vi "Ejercicio_basico_LabView.vi"() -> ()   [LabVIEW 2014]
uses:
  <vilib>/LabVIEW Interface for Arduino/Type Defs/Board Type.ctl
  <vilib>/LabVIEW Interface for Arduino/Type Defs/Pin Mode.ctl
  <vilib>/LabVIEW Interface for Arduino/LabVIEW Interface for Arduino.lvlib
panel:
  in  "VISA resource":refnum<visa-resource-name>
  in  "Boolean":bool
  in  "Board Type (Uno)":T1
  in  "Analog Input Pin (0)":u8
  in  "stop":bool
  out "Bomba":bool
  out "Vallvula":bool
  in  "Nivel Minimo":dbl
  in  "Nivel Maximo":dbl
  out "Alarma Bajo":bool
  out "Alarma Alto":bool
  out "Tank":dbl(slide) scale=0.0..100.0
  in  "Start":bool
  out "Sensor de nivel":dbl(slide) scale=0.0..100.0
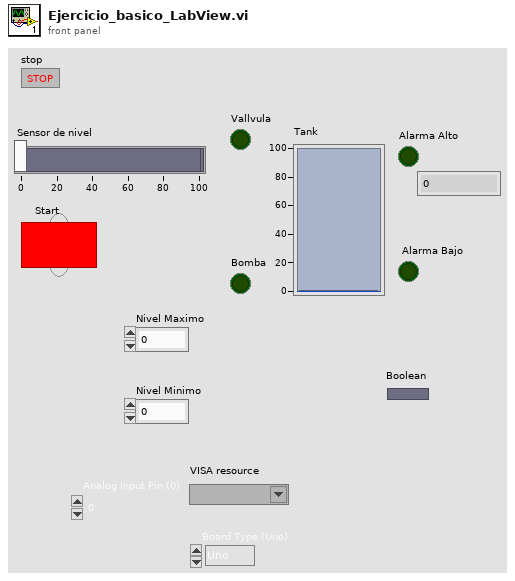
[diagram p1: front panel]
types:
  T1 = typedef "LabVIEW Interface for Arduino.lvlib/Board Type.ctl" = enum16{"Uno", "Dimuelanove w/Atmega 328", "Mega 2560"}
  T2 = typedef "LabVIEW Interface for Arduino.lvlib/Arduino Resource.ctl" = cluster{"VISA resource":refnum<visa-resource-name>, "Board Type":T1, "Connection Type":enum8{"USB / Serial"}, "Bytes Per Packet (15)":u8}
  T3 = typedef "LabVIEW Interface for Arduino.lvlib/Pin Mode.ctl" = enum8{"Input", "Output"}
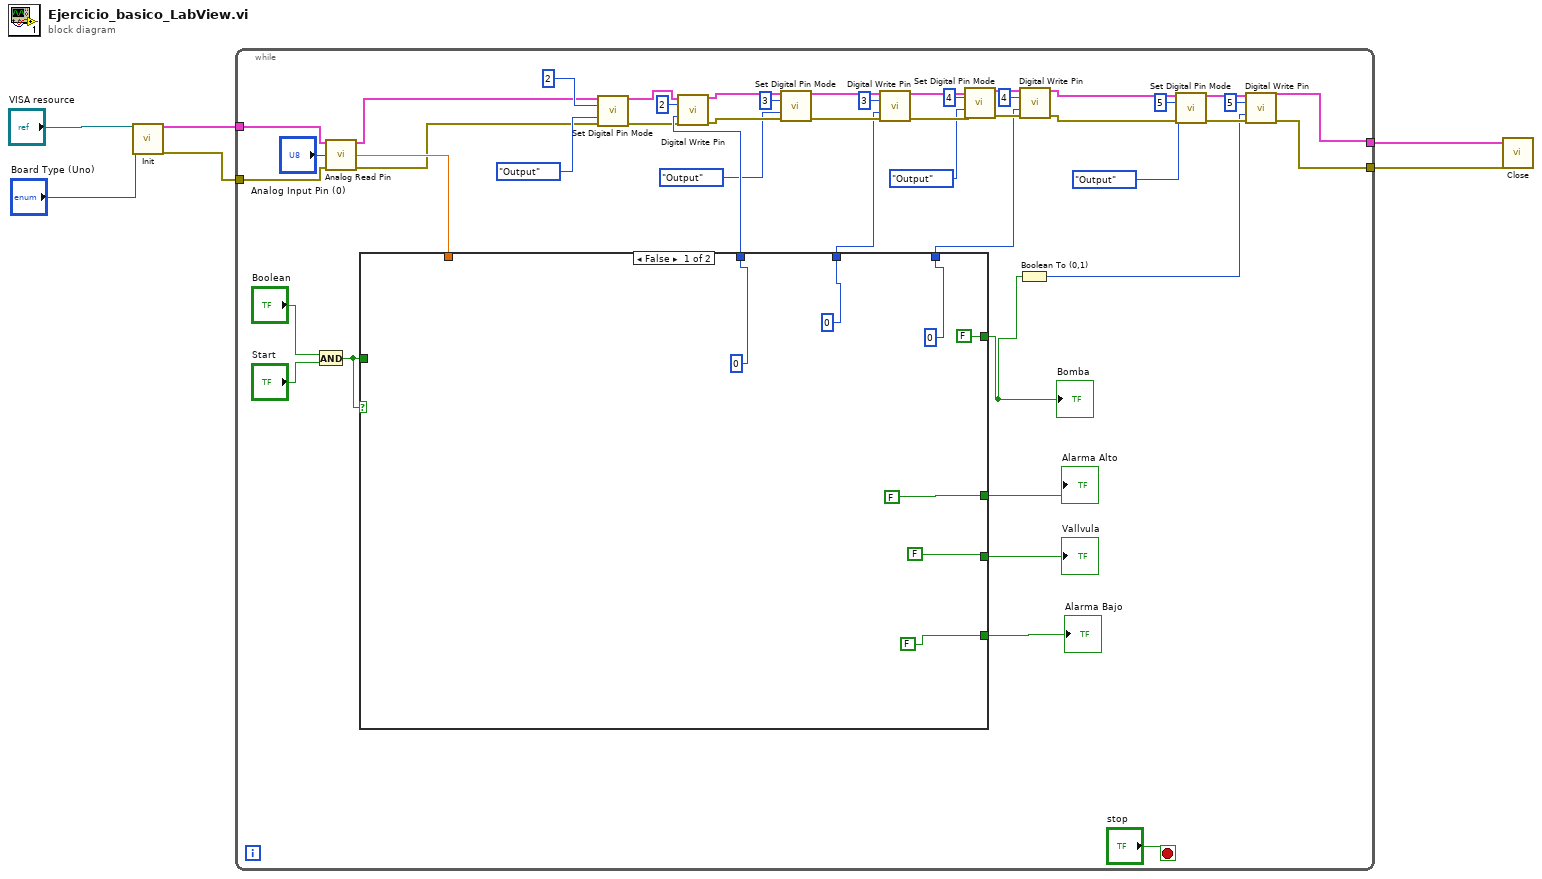
[diagram p0: block diagram]
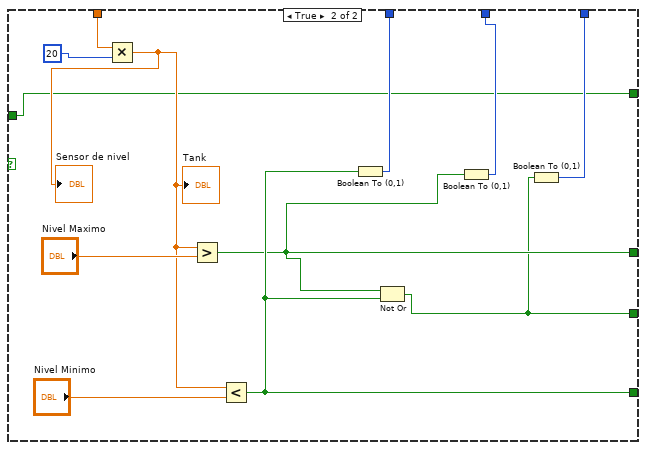
[diagram p2: hidden frame]
diagram:
  n1 = call <vilib>:"Init.vi"("VISA resource"="VISA resource", "Board Type (Uno)"="Board Type (Uno)") -> ("Arduino Resource"=w6:T2, "error out"=w4:errorcluster)  [unwired: 16 in]
  n2 = while {
    tunnel: w6 -> [w47]
    tunnel: [w15] -> w5
    tunnel: w4 -> [w46]
    tunnel: [w12] -> w3
    stop <- "stop" stop-if-true
    n3 = And(x="Boolean", y="Start") -> (x .and. y?=w18:bool)
    n4 = call <vilib>:"Analog Read Pin.vi"("Arduino Resource"=w47, "Analog Input Pin (0)"="Analog Input Pin (0)", "error in"=w46) -> ("Arduino Resource"=w40:T2, "Voltage"=w45:dbl, "error out"=w39:errorcluster)  [unwired: 10 in]
    n5 = case shown="False" w18 {
      tunnel: [FALSE w63] -> w51
      tunnel: [FALSE w66] -> w50
      tunnel: [FALSE w61] -> w49
      tunnel: w45 -> [_ w68]
      tunnel: [0 w65] -> w41
      tunnel: [0 w64] -> w29
      tunnel: [0 w62] -> w21
      tunnel: w18 -> [_ w60]
      tunnel: [FALSE w60] -> w7
      frame False {
      }
      frame True {
        n6 = Multiply(x=w68, y=20) -> (x*y=w67:dbl)
        "Sensor de nivel" <- w67
        "Tank" <- w67
        n7 = Greater?(x=w67, y="Nivel Maximo") -> (0:w63:bool)
        n8 = Less?(x=w67, y="Nivel Minimo") -> (x < y?=w66:bool)
        n9 = Boolean To (0,1)(Boolean=w66) -> (0, 1=w65:i16)
        n10 = Not Or(1:w66, 2:w63) -> (0:w61:bool)
        n11 = Boolean To (0,1)(Boolean=w63) -> (0, 1=w64:i16)
        n12 = Boolean To (0,1)(Boolean=w61) -> (0, 1=w62:i16)
      }
    }
    "Bomba" <- w7
    "Alarma Alto" <- w51
    "Alarma Bajo" <- w50
    "Vallvula" <- w49
    n13 = call <vilib>:"Set Digital Pin Mode.vi"("Arduino Resource"=w40, "Digital I/O Pin"=u8 2, "Pin Mode (Input)"=Pin_Mode."Output", "error in"=w39) -> ("Arduino Resource"=w38:T2, "error out"=w37:errorcluster)  [unwired: 10 in]
    n14 = call <vilib>:"Digital Write Pin.vi"("Arduino Resource"=w38, "Digital I/O Pin (0)"=u8 2, "Value (0)"=w41, "error in"=w37) -> ("Arduino Resource"=w36:T2, "error out"=w35:errorcluster)  [unwired: 10 in]
    n15 = call <vilib>:"Set Digital Pin Mode.vi"("Arduino Resource"=w36, "Digital I/O Pin"=u8 3, "Pin Mode (Input)"=Pin_Mode."Output", "error in"=w35) -> ("Arduino Resource"=w33:T2, "error out"=w32:errorcluster)  [unwired: 10 in]
    n16 = call <vilib>:"Digital Write Pin.vi"("Arduino Resource"=w33, "Digital I/O Pin (0)"=u8 3, "Value (0)"=w29, "error in"=w32) -> ("Arduino Resource"=w25:T2, "error out"=w26:errorcluster)  [unwired: 10 in]
    n17 = call <vilib>:"Set Digital Pin Mode.vi"("Arduino Resource"=w25, "Digital I/O Pin"=u8 4, "Pin Mode (Input)"=Pin_Mode."Output", "error in"=w26) -> ("Arduino Resource"=w28:T2, "error out"=w27:errorcluster)  [unwired: 10 in]
    n18 = Boolean To (0,1)(Boolean=w7) -> (0, 1=w8:i16)
    n19 = call <vilib>:"Digital Write Pin.vi"("Arduino Resource"=w28, "Digital I/O Pin (0)"=u8 4, "Value (0)"=w21, "error in"=w27) -> ("Arduino Resource"=w17:T2, "error out"=w14:errorcluster)  [unwired: 10 in]
    n20 = call <vilib>:"Set Digital Pin Mode.vi"("Arduino Resource"=w17, "Digital I/O Pin"=u8 5, "Pin Mode (Input)"=Pin_Mode."Output", "error in"=w14) -> ("Arduino Resource"=w16:T2, "error out"=w13:errorcluster)  [unwired: 10 in]
    n21 = call <vilib>:"Digital Write Pin.vi"("Arduino Resource"=w16, "Digital I/O Pin (0)"=u8 5, "Value (0)"=w8, "error in"=w13) -> ("Arduino Resource"=w15:T2, "error out"=w12:errorcluster)  [unwired: 10 in]
  }
  n22 = call <vilib>:"Close.vi"("Arduino Resource"=w5, "error in"=w3) -> ()  [unwired: 13 in, 1 out]
